vi "upgrade_capacitor.vi"(7 "Quantity 2":string, 8 "Fault type (phases)":string="BC", 9 "Capacitores":string="  N0083A                   0.001 .0001  36.8                                   0\n  N0083B                   0.001 .0001  36.8                                   0\n  N0083C                   0.001 .0001  36.8                                   0\n  N0088A                   0.001 .0001   9.2                                   0\n  N0090B                   0.001 .0001   9.2                                   0\n  N0092C                   0.001 .0001   9.2                                   0", 10 "Event type":string="CL", 11 "Node":string="83") -> (1 "Actual caps":string)   [LabVIEW 2020]
panel:
  out "F-format string 2":string
  out "F-format string":string
  in  "Snubber":bool
  # "FRAÇÃO DE POTÊNCIA (%) - diferente das cargas"
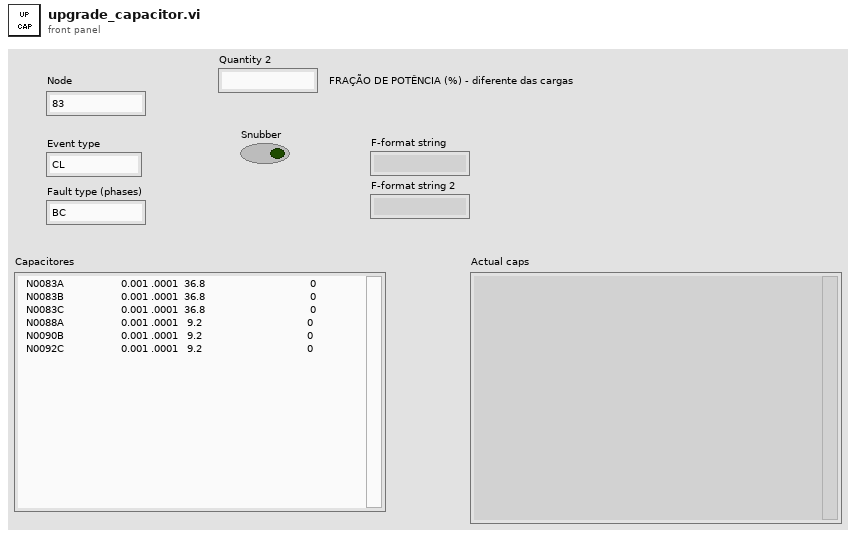
[diagram p1: front panel]
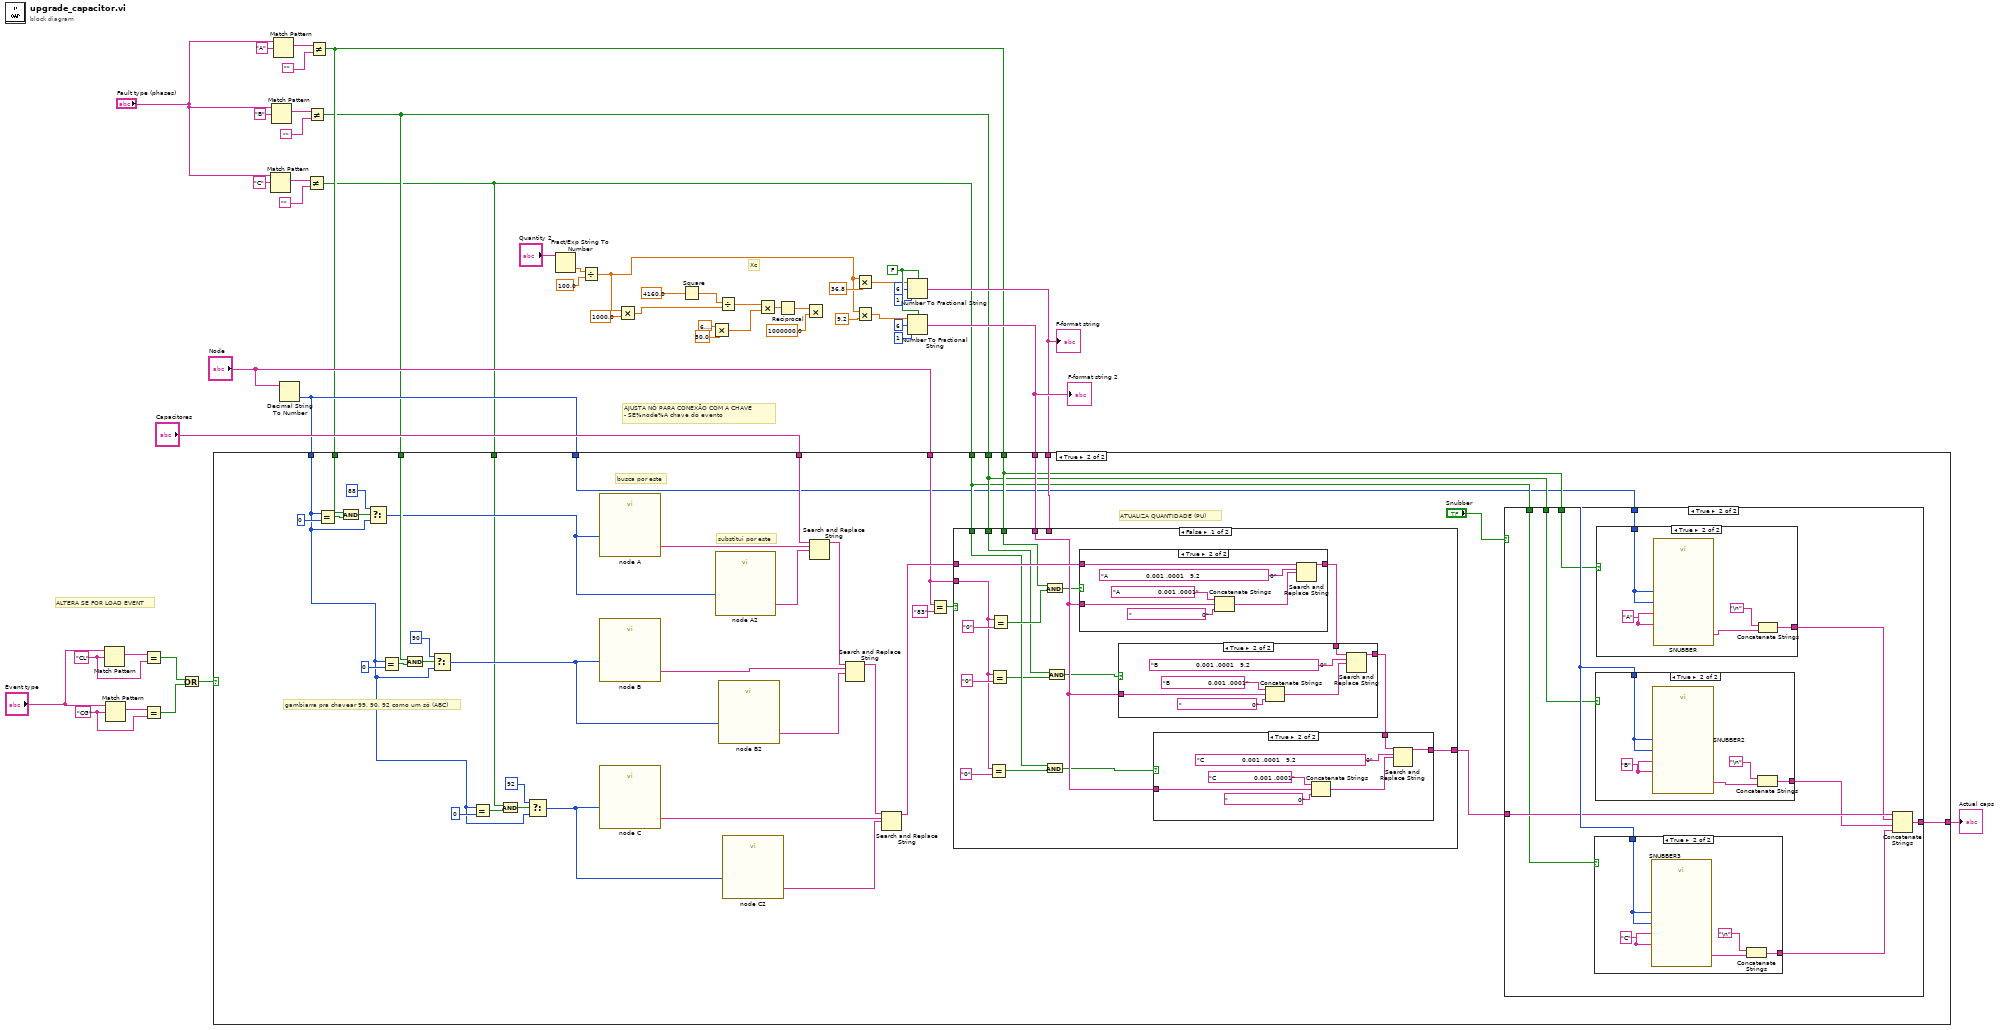
[diagram p0: block diagram]
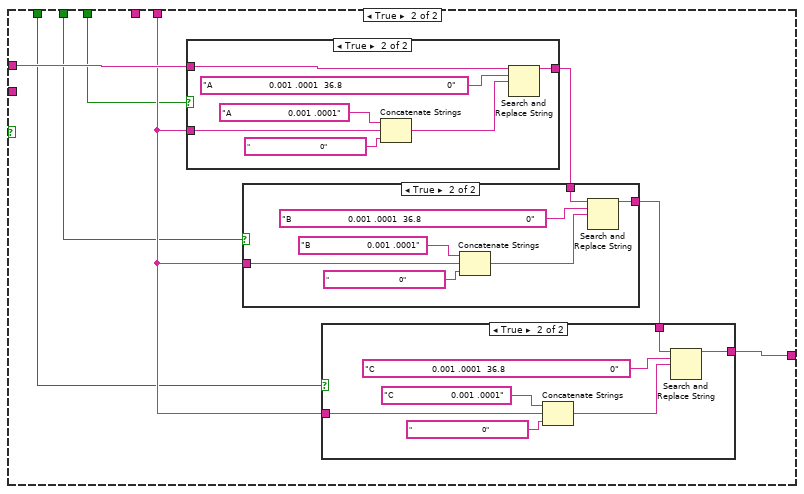
[diagram p6: hidden frame]
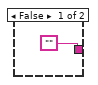
[diagram p11: hidden frame]
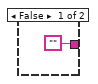
[diagram p12: hidden frame]
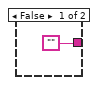
[diagram p13: hidden frame]
diagram:
  w31 = FALSE ("use system decimal point (T)")
  w49 = "CL" ("regular expression")
  w47 = "CG" ("regular expression")
  # "Xc"
  # "ALTERA SE FOR LOAD EVENT"
  # "AJUSTA NÓ PARA CONEXÃO COM A CHAVE\n- SE%node%A chave do evento"
  n1 = Match Pattern(string="Event type", regular expression=w49) -> (match substring=w48:string)  [unwired: 1 in, 3 out]
  n2 = Match Pattern(string="Event type", regular expression=w47) -> (match substring=w50:string)  [unwired: 1 in, 3 out]
  n3 = Equal?(x=w48, y=w49) -> (x = y?=w45:bool)
  n4 = Equal?(x=w50, y=w47) -> (x = y?=w46:bool)
  n5 = Or(x=w45, y=w46) -> (x .or. y?=w44:bool)
  n6 = Match Pattern(string="Fault type (phases)", regular expression="C") -> (match substring=w35:string)  [unwired: 1 in, 3 out]
  n7 = Match Pattern(string="Fault type (phases)", regular expression="B") -> (match substring=w38:string)  [unwired: 1 in, 3 out]
  n8 = Match Pattern(string="Fault type (phases)", regular expression="A") -> (match substring=w41:string)  [unwired: 1 in, 3 out]
  n9 = Decimal String To Number(string="Node") -> (number=w4:i32)  [unwired: 2 in, 1 out]
  n10 = Not Equal?(x=w35, y="") -> (x != y?=w1:bool)
  n11 = Not Equal?(x=w38, y="") -> (x != y?=w2:bool)
  n12 = Not Equal?(x=w41, y="") -> (x != y?=w3:bool)
  n13 = Fract/Exp String To Number(string="Quantity 2") -> (number=w8:dbl)  [unwired: 3 in, 1 out]
  n14 = Divide(x=w8, y=100.0) -> (x/y=w5:dbl)
  n15 = Multiply(x=w5, y=1000.0) -> (x*y=w13:dbl)
  n16 = Square(x=4160.0) -> (x^2=w22:dbl)
  n17 = Multiply(x=6.283185307179586, y=50.0) -> (x*y=w18:dbl)
  n18 = Divide(x=w22, y=w13) -> (x/y=w19:dbl)
  n19 = Multiply(x=w19, y=w18) -> (x*y=w17:dbl)
  n20 = Reciprocal(x=w17) -> (1/x=w15:dbl)
  n21 = Multiply(x=w15, y=1000000.0) -> ()  [unwired: 1 out]
  n22 = Multiply(x=w5, y=36.8) -> (x*y=w11:dbl)
  n23 = Multiply(x=w5, y=9.2) -> (x*y=w9:dbl)
  n24 = Number To Fractional String(use system decimal point (T)=w31, number=w11, width (-)=i16 6, precision (6)=i16 1) -> (F-format string=w29:string)
  "F-format string" <- w29
  n25 = Number To Fractional String(use system decimal point (T)=w31, number=w9, width (-)=i16 6, precision (6)=i16 1) -> (F-format string=w30:string)
  "F-format string 2" <- w30
  n26 = case shown="True" w44 {
    tunnel: "Capacitores" -> [w52 w88]
    tunnel: [w52 w84] -> w32
    tunnel: w4 -> [_ w67]
    tunnel: w3 -> [_ w75]
    tunnel: w2 -> [_ w74]
    tunnel: w1 -> [_ w73]
    tunnel: w30 -> [_ w77]
    tunnel: w29 -> [_ w81]
    tunnel: "Node" -> [_ w76]
    tunnel: w4 -> [_ w54]
    tunnel: w3 -> [_ w69]
    tunnel: w2 -> [_ w58]
    tunnel: w1 -> [_ w53]
    frame False {
    }
    frame True {
      # "gambiarra pra chavear 99, 90, 92 como um só (ABC)"
      # "ATUALIZA QUANTIDADE (PU)"
      # "substitui por este"
      # "busca por este"
      n27 = Equal?(x=w54, y=0) -> (x = y?=w70:bool)
      n28 = And(x=w69, y=w70) -> (x .and. y?=w68:bool)
      n29 = Select(t=88, s=w68, f=w54) -> (s? t:f=w57:i32)
      n30 = Equal?(x=w54, y=0) -> (x = y?=w64:bool)
      n31 = And(x=w58, y=w64) -> (x .and. y?=w63:bool)
      n32 = Select(t=90, s=w63, f=w54) -> (s? t:f=w55:i32)
      n33 = Equal?(x=w54, y=0) -> (x = y?=w60:bool)
      n34 = And(x=w53, y=w60) -> (x .and. y?=w59:bool)
      n35 = Select(t=92, s=w59, f=w54) -> (s? t:f=w56:i32)
      n36 = call "node A"("node"=w57) -> ("Result"=w87:string)  [unwired: 13 in, 1 out]
      n37 = call "node B"("node"=w55) -> ("Result"=w85:string)  [unwired: 13 in, 1 out]
      n38 = call "node C"("node"=w56) -> ("Result"=w93:string)  [unwired: 13 in, 1 out]
      n39 = call "node A2"("node"=w57) -> ("Result"=w91:string)  [unwired: 13 in, 1 out]
      n40 = call "node B2"("node"=w55) -> ("Result"=w90:string)  [unwired: 13 in, 1 out]
      n41 = call "node C2"("node"=w56) -> ("Result"=w89:string)  [unwired: 13 in, 1 out]
      n42 = Search and Replace String(input string=w88, search string=w87, replace string=w91) -> (result string=w86:string)  [unwired: 5 in, 3 out]
      n43 = Search and Replace String(input string=w86, search string=w85, replace string=w90) -> (result string=w92:string)  [unwired: 5 in, 3 out]
      n44 = Search and Replace String(input string=w92, search string=w93, replace string=w89) -> (result string=w82:string)  [unwired: 5 in, 3 out]
      n45 = Equal?(x=w76, y="83") -> (x = y?=w79:bool)
      n46 = case shown="False" w79 {
        tunnel: w82 -> [w109 w143]
        tunnel: w81 -> [_ w140]
        tunnel: [w106 w139] -> w80
        tunnel: w77 -> [w102 _]
        tunnel: w76 -> [w104 _]
        tunnel: w75 -> [w100 w138]
        tunnel: w74 -> [w99 w137]
        tunnel: w73 -> [w96 w136]
        frame False {
          n47 = Equal?(x=w104, y="0") -> (x = y?=w98:bool)
          n48 = Equal?(x=w104, y="0") -> (x = y?=w95:bool)
          n49 = Equal?(x=w104, y="0") -> (x = y?=w103:bool)
          n50 = And(x=w100, y=w103) -> (x .and. y?=w101:bool)
          n51 = And(x=w96, y=w98) -> (x .and. y?=w97:bool)
          n52 = And(x=w99, y=w95) -> (x .and. y?=w94:bool)
          n53 = case shown="True" w101 {
            tunnel: [w128 w131] -> w111
            tunnel: w102 -> [_ w130]
            tunnel: w109 -> [w128 w129]
            frame False {
            }
            frame True {
              n54 = Concatenate Strings("A                   0.001 .0001", w130, "                                   0") -> (w132:string)
              n55 = Search and Replace String(input string=w129, search string="A                   0.001 .0001   9.2                                   0", replace string=w132) -> (result string=w131:string)  [unwired: 5 in, 3 out]
            }
          }
          n56 = case shown="True" w94 {
            tunnel: w111 -> [w120 w123]
            tunnel: [w120 w122] -> w110
            tunnel: w102 -> [_ w121]
            frame False {
            }
            frame True {
              n57 = Concatenate Strings("B                   0.001 .0001", w121, "                                   0") -> (w124:string)
              n58 = Search and Replace String(input string=w123, search string="B                   0.001 .0001   9.2                                   0", replace string=w124) -> (result string=w122:string)  [unwired: 5 in, 3 out]
            }
          }
          n59 = case shown="True" w97 {
            tunnel: w110 -> [w112 w115]
            tunnel: w102 -> [_ w114]
            tunnel: [w112 w113] -> w106
            frame False {
            }
            frame True {
              n60 = Concatenate Strings("C                   0.001 .0001", w114, "                                   0") -> (w116:string)
              n61 = Search and Replace String(input string=w115, search string="C                   0.001 .0001   9.2                                   0", replace string=w116) -> (result string=w113:string)  [unwired: 5 in, 3 out]
            }
          }
        }
        frame True {
          n62 = case shown="True" w138 {
            tunnel: w143 -> [w160 w167]
            tunnel: [w160 w162] -> w142
            tunnel: w140 -> [_ w161]
            frame False {
            }
            frame True {
              n63 = Concatenate Strings("A                   0.001 .0001", w161, "                                   0") -> (w163:string)
              n64 = Search and Replace String(input string=w167, search string="A                   0.001 .0001  36.8                                   0", replace string=w163) -> (result string=w162:string)  [unwired: 5 in, 3 out]
            }
          }
          n65 = case shown="True" w137 {
            tunnel: w142 -> [w152 w155]
            tunnel: [w152 w154] -> w141
            tunnel: w140 -> [_ w153]
            frame False {
            }
            frame True {
              n66 = Concatenate Strings("B                   0.001 .0001", w153, "                                   0") -> (w156:string)
              n67 = Search and Replace String(input string=w155, search string="B                   0.001 .0001  36.8                                   0", replace string=w156) -> (result string=w154:string)  [unwired: 5 in, 3 out]
            }
          }
          n68 = case shown="True" w136 {
            tunnel: w141 -> [w144 w147]
            tunnel: w140 -> [_ w146]
            tunnel: [w144 w145] -> w139
            frame False {
            }
            frame True {
              n69 = Concatenate Strings("C                   0.001 .0001", w146, "                                   0") -> (w148:string)
              n70 = Search and Replace String(input string=w147, search string="C                   0.001 .0001  36.8                                   0", replace string=w148) -> (result string=w145:string)  [unwired: 5 in, 3 out]
            }
          }
        }
      }
      n71 = case shown="True" "Snubber" {
        tunnel: w67 -> [_ w177]
        tunnel: w80 -> [w168 w176]
        tunnel: [w168 w172] -> w84
        tunnel: w75 -> [_ w171]
        tunnel: w74 -> [_ w170]
        tunnel: w73 -> [_ w169]
        frame False {
        }
        frame True {
          n72 = case shown="True" w169 {
            tunnel: w177 -> [_ w183]
            tunnel: ["" w179] -> w173
            frame False {
            }
            frame True {
              w182 = "C"
              n73 = call "SNUBBER3"("phase_out"=w182, "node_in"=w183, "phase_in"=w182, "node_out"=w183) -> ("Result"=w180:string)  [unwired: 10 in, 1 out]
              n74 = Concatenate Strings("\n", w180) -> (w179:string)
            }
          }
          n75 = case shown="True" w170 {
            tunnel: w177 -> [_ w189]
            tunnel: ["" w185] -> w174
            frame False {
            }
            frame True {
              w188 = "B"
              n76 = call "SNUBBER2"("phase_out"=w188, "node_in"=w189, "phase_in"=w188, "node_out"=w189) -> ("Result"=w186:string)  [unwired: 10 in, 1 out]
              n77 = Concatenate Strings("\n", w186) -> (w185:string)
            }
          }
          n78 = case shown="True" w171 {
            tunnel: w177 -> [_ w195]
            tunnel: ["" w191] -> w175
            frame False {
            }
            frame True {
              w194 = "A"
              n79 = call "SNUBBER"("phase_out"=w194, "node_in"=w195, "phase_in"=w194, "node_out"=w195) -> ("Result"=w192:string)  [unwired: 10 in, 1 out]
              n80 = Concatenate Strings("\n", w192) -> (w191:string)
            }
          }
          n81 = Concatenate Strings(w176, w175, w174, w173) -> (w172:string)
        }
      }
    }
  }
  "Actual caps" <- w32
